vi "Autofocus.vi"(8 "error in":errorcluster, 11 "controller in":refnum<k24>) -> (0 "error out":errorcluster, 3 "Image Out 2":T1(plugin-control))   [LabVIEW 2011]
uses:
  C:/Users/Admin/Desktop/Gantry Code Transfer/source/Code Transfer/Aerotech.A3200.dll
  Aerotech.A3200.dll
  <vilib>/vision/NI_Vision_Development_Module.lvlib
  <vilib>/vision/driver/NI_Vision_Acquisition_Software.lvlib
panel:
  out "Done moving?":bool
  out "Current pos?":dbl[](array[numeric])
  out "Z hieghts":dbl[](array[numeric])
  out "intensities":dbl[](array[numeric])
  out "Max Intensity":dbl
  out "ZMAX":dbl
  out "Waveform Chart":sgl(graph)
  out "Numeric":dbl
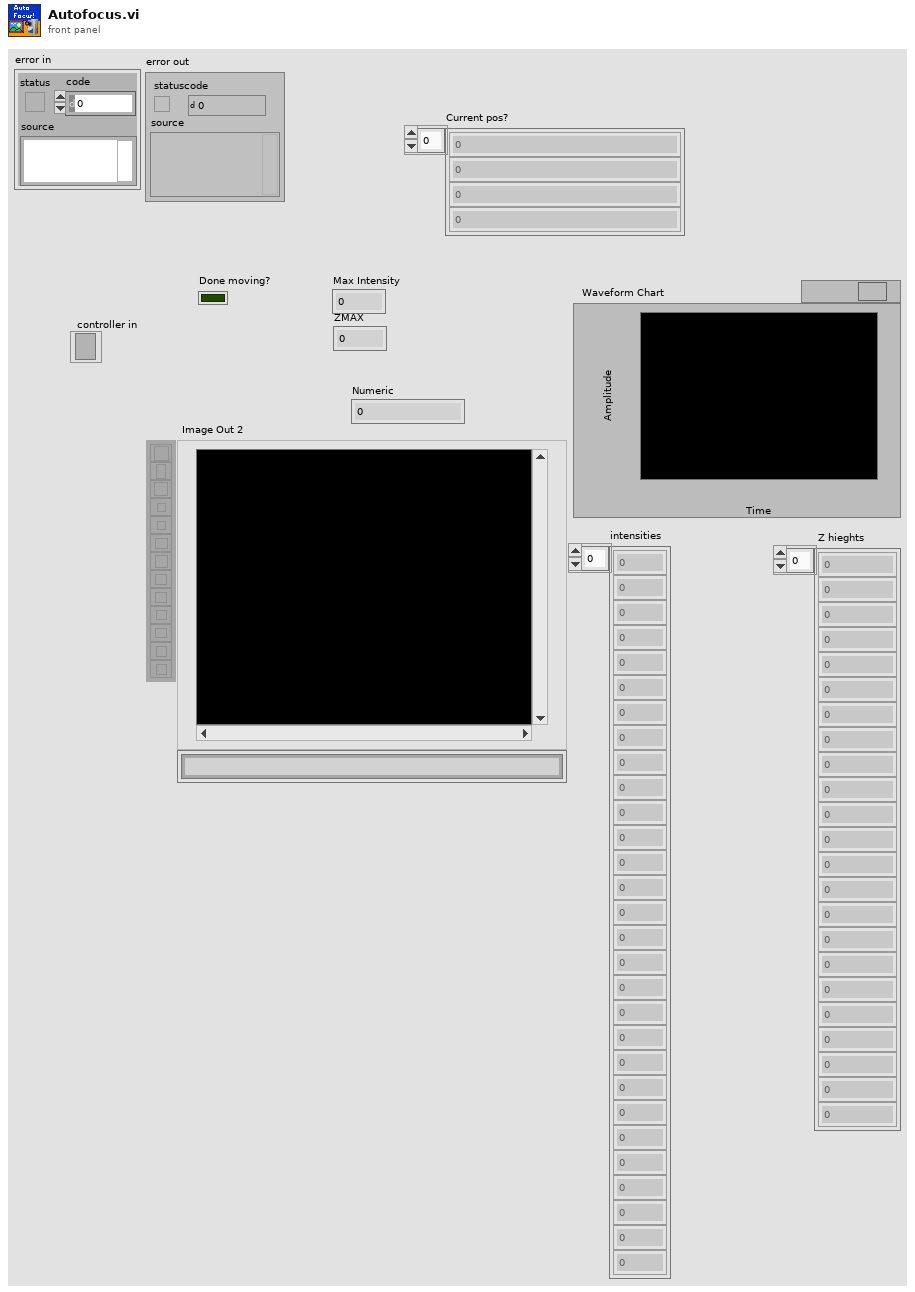
[diagram p1: front panel]
types:
  T1 = typedef "IMAQ Image.ctl" = refnum<image>
  T2 = typedef "Image Type" = u32
  T3 = typedef "IMAQdx.ctl" = refnum<k21>
  T4 = typedef "IMAQ Rectangle" = cluster{"Left":i32, "Top":i32, "Right":i32, "Bottom":i32, "Rotation":dbl}
  T5 = typedef "IMAQ Point" = cluster{"X":sgl, "Y":sgl}
  T6 = cluster{"Mean Intensity":sgl, "Standard  Deviation":sgl, "Minimum Intensity":sgl, "Maximum Intensity":sgl}
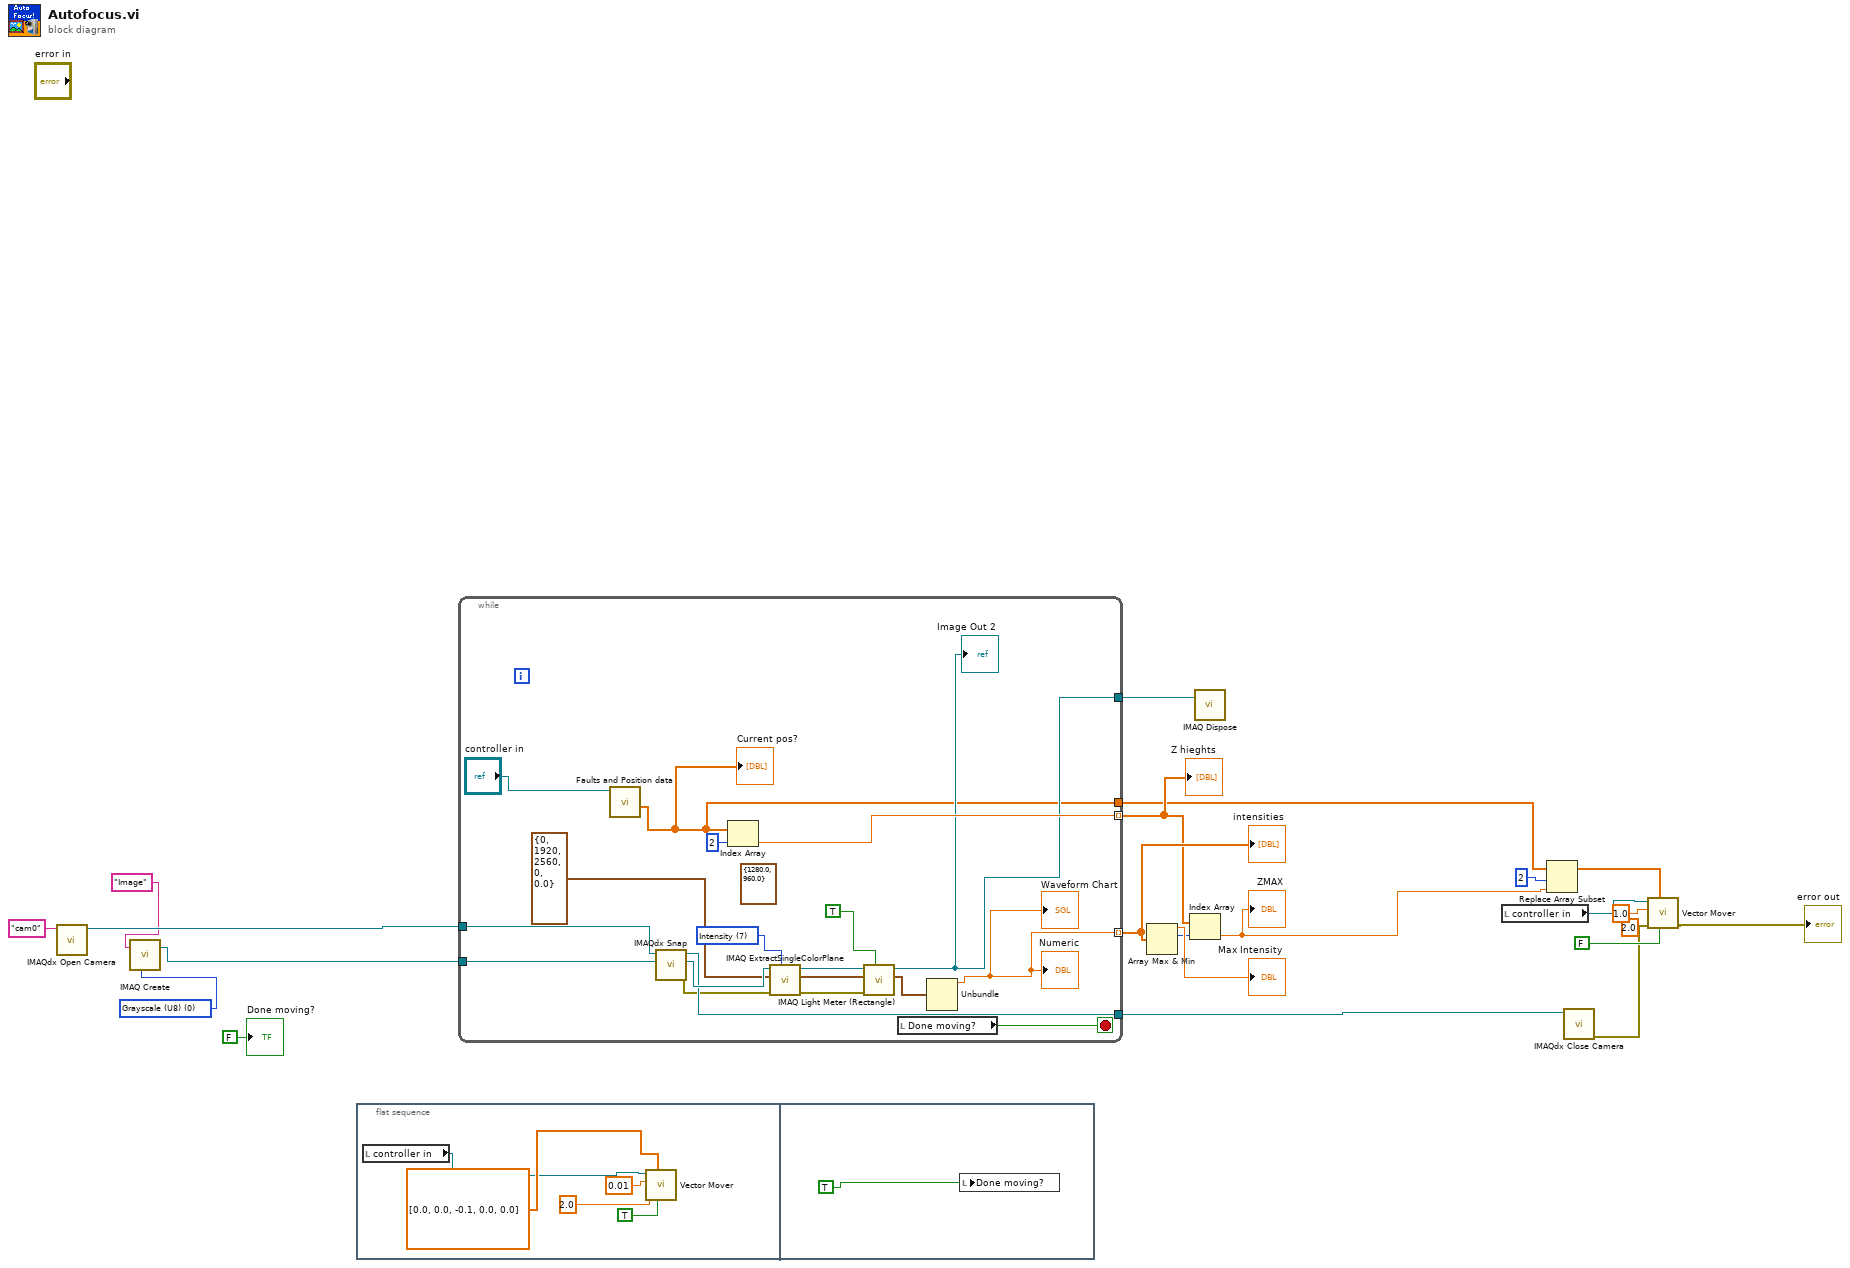
[diagram p0: block diagram]
diagram:
  w9 = T2 0 items=["Grayscale (U8)", "Grayscale (I16)", "Grayscale (SGL)", "Complex (CSG)", "RGB (U32)", "HSL (U32)", "RGB (U64)", "Grayscale (U16)"] ("Image Type")
  n1 = call <vilib>:"IMAQdx Open Camera.vi"("Session In"="cam0" ("Interface Name")) -> ("Session Out"=w10:T3)  [unwired: 9 in, 1 out]
  n2 = call "IMAQ Create"("Image Name"="Image", "Image Type"=w9) -> ("New Image"=w7:T1)  [unwired: 3 in, 1 out]
  n3 = flat-sequence {
    frame #0 {
      n4 = local read "controller in"() -> (w26:refnum<k24>)
      n5 = call "Vector Mover.vi"("Absolute/Relative (F/T)"=TRUE, "Movement Vector"=dbl[] [0.0, 0.0, -0.1, 0.0, 0.0], "Angular Speed"=2.0, "Vector Speed"=0.01, "controller in"=w26) -> ()  [unwired: 1 in, 4 out]
    }
    frame #1 {
      n6 = local write "Done moving?"(TRUE ("Done moving?")) -> ()
    }
  }
  n7 = while {
    tunnel: [w29] -> w22 mode=indexing
    tunnel: [w41] -> w5 mode=indexing
    tunnel: [w37] -> w14
    tunnel: [w39] -> w12
    tunnel: w10 -> [w35]
    tunnel: w7 -> [w36]
    tunnel: [w33] -> w4
    stop <- w32 stop-if-true
    (unwired) T5 {"X"=1280.0, "Y"=960.0} ("Point")
    w45 = 7 items=["Red", "Green", "Blue", "Hue", "Saturation", "Luminance", "Value", "Intensity"] ("Color Plane")
    n8 = call "Faults and Position data.vi"("Controller In"="controller in") -> ("Positions"=w33:dbl[])  [unwired: 7 in, 3 out]
    "Current pos?" <- w33
    n9 = call <vilib>:"IMAQdx Snap.vi"("Image In"=w36, "Session In"=w35) -> ("error out"=w38:errorcluster, "Image Out"=w40:T1, "Session Out"=w39:T3)  [unwired: 7 in]
    n10 = Index Array(array=w33, index=2) -> (element=w41:dbl)
    n11 = call "IMAQ ExtractSingleColorPlane"("Color Plane"=w45, "error in (no error)"=w38, "Image Src"=w40) -> ("error out"=w44:errorcluster, "Image Dst Out"=w43:T1)  [unwired: 7 in]
    n12 = call "IMAQ Light Meter (Rectangle)"("Show Search Area"=TRUE, "error in (no error)"=w44, "Rectangle"=T4 {"Left"=0, "Top"=1920, "Right"=2560, "Bottom"=0, "Rotation"=0.0}, "Image"=w43) -> ("Gray Level Intensities"=w30:T6, "Image Out"=w37:T1)  [unwired: 3 in, 3 out]
    "Image Out 2" <- w37
    n13 = local read "Done moving?"() -> (w32:bool)
    n14 = Unbundle(w30) -> ("Mean Intensity"=w29:sgl)  [unwired: 3 out]
    "Waveform Chart" <- w29
    "Numeric" <- w29
  }
  "intensities" <- w22
  "Z hieghts" <- w5
  n15 = Array Max & Min(array=w22) -> (max value=→"Max Intensity":sgl, max index (indices)=w20:i32)  [unwired: 2 out]
  n16 = Index Array(array=w5, index=w20) -> (element=w3:dbl)
  "ZMAX" <- w3
  n17 = call "IMAQ Dispose"("Image"=w14) -> ()  [unwired: 5 in, 1 out]
  n18 = local read "controller in"() -> (w15:refnum<k24>)
  n19 = Replace Array Subset(array=w4, new element=w3, index=2) -> (w2:dbl[])
  n20 = call <vilib>:"IMAQdx Close Camera.vi"("Session In"=w12) -> ("error out"=w11:errorcluster)  [unwired: 10 in]
  n21 = call "Vector Mover.vi"("Absolute/Relative (F/T)"=FALSE, "Movement Vector"=w2, "error in (no error)"=w11, "Angular Speed"=2.0, "Vector Speed"=1.0, "controller in"=w15) -> ("error out"=→"error out":errorcluster)  [unwired: 3 out]
  "Done moving?" <- FALSE ("Done moving?")
